vi "testing -- App - RUS scan V2.vi"(4 "Bypass error dialog":bool=TRUE, 5 "saved frequency unit":bool=TRUE, 6 "Zero amplitude at the end":bool, 7 "Save data settings":T3={"Save data"=TRUE, "Data Root Path"=path "C:/data/RUS/Experiment/ProbeTest/Probe10/YBCO_3/sweep4", "File Prefix"="289.47200K_1400_3000_", "File Format"=enum."BINARY", "Save column names"=FALSE, "File Comments"="<Description of the current file>\r\nColumns:Frequency\\tX\\tY\r\n    ITC Temp= 299.200000\r\n    LTC Temp= 0.000000\r\n          ITC_set=295.00000\r\n", "User/Prj"="<User Name/Project Description>"}, 8 "error in (no error)":errorcluster, 9 "Fast swep settings":T1={"Update rate (Hz)"=250.0, "Start F, Hz"=1400000.0, "Stop F"=3000000.0, "Number of points"=6000, "Amplitude"=2.1, "Init&amplitude"=TRUE, "IF"=1000.0, "Time constant"=0.003} {"IF" format="%#_6p"; "Amplitude" min=0.0 max=2.5; "Number of points" format="%.0p"; "Stop F" format="%#_6p"; "Start F, Hz" format="%#_6p"; "Update rate (Hz)" format="%0.2f"}, 11 "Lock-in DAQ settings":T2={"Lockin mode"=enum."NI-DAQ", "DAQmx Device"="Dev1", "SR Lockin"="GPIB0::10::INSTR", "Clock Multiplier"=64, "Low-pass filter"=enum."No filtering", "Ranges and couplings "=[{"Range"=2.5, "Coupling"=10106}], "Samples per read"=10, "Record IF"=FALSE, "Auto-phase"=FALSE} {"Ranges and couplings"."Coupling" items=["default"=-1, "RSE"=10083, "NRSE"=10078, "Differential"=10106, "Pseudodifferential"=12529]}) -> (0 "error out":errorcluster, 2 "Actual file path":path=path "C:/data/RUS/Experiment/ProbeTest/Probe10/YBCO_3/sweep4/February_2012/020712/289.73300K_1400_3000_001_020712.bin")   [LabVIEW 2010]
uses:
  <vilib>/Utility/error.llb/DialogType.ctl
  C:/Program Files (x86)/National Instruments/LabVIEW 2010/resource/objmgr/daqmx.rc
  RUS/Controls/Sweep settings.ctl
  RUS/Controls/Lock-in DAQ settings.ctl
  File/Controls/File formats.ctl
  File/Controls/Save data settings.ctl
  single sweep - adaptive parameters.ctl
  single sweep - frequency chunks.ctl
  wavepacket.ctl
  cursor winow.ctl
  next chunk -- parameters.ctl
  find peak -- parameters.ctl
panel:
  in  "Tab : everything":enum32{"main", "everything else", "adaptive"}(tab)=enum."adaptive"
  in  "complex plane scale gauge":dbl(slide)=0.07327431522473847 caption="Volts" scale=0.0001..0.1
  in  "show plot pallets":bool
  in  "highlight last # sec":dbl=4.0
  out "Plot:response":cluster{dbl[], dbl[]}[](graph)
  out "Plot:complex plane":cluster{dbl[], dbl[]}[](graph)
  in  "Tab : sweep controls":enum32{"Main controls", "File", "Advanced"}(tab)
  in  "Manual\nPhase":dbl(slide) scale=-180.0..180.0
  out "Error status byte\n(bit 5 - FAST aborted)":u8 format="%08b"
  out "STD status byte":u8 format="%08b"
  out "DO array  making time":u32=3
  out "DO write time, ms":u32=44
  out "Loop counter":i32=599
  out "Pre-sweep delay, s":dbl=0.2
  out "Samples in buffer":u32
  out "Actual setup time, ms":u32=1470
  in  "progress (sec)":dbl(slide)=0.20199999981559813 caption="seconds" min=80.0 max=80.0 scale=0.0..24.0
  in  "Plot when running":bool
  in  "algorithm":string="uniform"
  in  "Graph update rate, ms":u32=30
  in  "stop":bool
  out "Progress, %":u8(slide)=1 scale=0.0..100.0
  in  "cursor bracket: Scan, win":T5={"left"=1402.9280000000003, "right "=1414.9280000000003, "center"=1408.9280000000003, "window"=12.0, "cursors"=[1, 2, 3], "relative"=1, "absolute"=4, "fixed vertical offset"=2421.6740576496672, "vertical offset"=2421.6740576496672, "skew"=0.0, "default window frac"=0.0, "kind"=enum."symmetric", "skew.left"=0.5, "skew.right"=0.0, "Plot ref"=refnum, "wing order"=enum."back"}
  out "fancy circles":cluster{dbl[], dbl[]}[](array[cluster])=[{[0.004347976639836461, 0.0043237329011621035, 0.004251384023380436, 0.004132070991513198, 0.003967675443347089, 0.0037607899948818246, 0.0035146773532270816, 0.00323321886176232, 0.0029208532890330928, 0.002582506826719488, 0.00222351540065057, 0.0018495405200665291, 0.0014664799922359413, 0.001080374910511962, 0.0006973143826813736, 0.0003233395020973332, -3.56519239715844e-05, -0.0003739983862851902, -0.0006863639590144167, -0.0009678224504791784, -0.0012139350921339205, -0.0014208205405991845, -0.001585216088765295, -0.0017045291206325324, -0.0017768779984142003, -0.001801121737088557, -0.0017768779984142003, -0.0017045291206325324, -0.0015852160887652941, -0.001420820540599184, -0.00121393509213392, -0.000967822450479178, -0.0006863639590144162, -0.00037399838628518847, -3.5651923971582664e-05, 0.0003233395020973332, 0.0006973143826813741, 0.0010803749105119625, 0.0014664799922359426, 0.001849540520066531, 0.0022235154006505697, 0.002582506826719488, 0.0029208532890330936, 0.003233218861762321, 0.003514677353227083, 0.0037607899948818254, 0.003967675443347089, 0.004132070991513199, 0.004251384023380437, 0.0043237329011621035], [-0.00253283204245687, -0.0021474888509143563, -0.001768222751695333, -0.0014010149977470693, -0.0010516566747086093, -0.0007256573720308159, -0.00042815829345946126, -0.00016385117718095135, 6.309569569158376e-05, 0.0002491032374014545, 0.0003912379979003752, 0.0004872584271080889, 0.0005356502254961651, 0.0005356502254961651, 0.00048725842710808844, 0.0003912379979003752, 0.00024910323740145405, 6.309569569158376e-05, -0.00016385117718095135, -0.0004281582934594617, -0.0007256573720308154, -0.0010516566747086097, -0.00140101499774707, -0.0017682227516953328, -0.0021474888509143567, -0.002532832042456871, -0.002918175233999384, -0.003297441333218408, -0.003664649087166672, -0.004014007410205131, -0.004340006712882925, -0.004637505791454279, -0.004901812907732789, -0.005128759780605325, -0.005314767322315195, -0.005456902082814115, -0.0055529225120218295, -0.005601314310409906, -0.005601314310409906, -0.005552922512021829, -0.005456902082814115, -0.005314767322315195, -0.0051287597806053235, -0.004901812907732788, -0.004637505791454277, -0.004340006712882922, -0.004014007410205131, -0.0036646490871666704, -0.0032974413332184063, -0.0029181752339993822]}, {[-0.0007985969840225416, -0.0005913945404828922, -0.0003841920969432428, -0.0001769896534035934, 3.0212790136055923e-05, 0.00023741523367570524, 0.0004446176772153548, 0.0006518201207550041, 0.0008590225642946534, 0.0010662250078343027, 0.001273427451373952, 0.0014806298949136016, 0.001687832338453251, 0.0018950347819929002, 0.00210223722553255, 0.0023094396690721986, 0.002516642112611848, 0.0027238445561514977, 0.0029310469996911472, 0.003138249443230796], [-0.004804300169328853, -0.004577153356641655, -0.004350006543954456, -0.004122859731267258, -0.00389571291858006, -0.0036685661058928616, -0.003441419293205663, -0.003214272480518465, -0.0029871256678312666, -0.002759978855144068, -0.00253283204245687, -0.0023056852297696716, -0.002078538417082473, -0.0018513916043952751, -0.0016242447917080766, -0.0013970979790208786, -0.0011699511663336801, -0.0009428043536464817, -0.0007156575409592832, -0.0004885107282720852]}, {[-0.0009980406754980312, -0.0007708938628108329, -0.0005437470501236345, -0.0003166002374364362, -8.945342474923792e-05, 0.00013769338793796033, 0.0003648402006251588, 0.0005919870133123571, 0.0008191338259995553, 0.0010462806386867538, 0.0012734274513739518, 0.0015005742640611503, 0.0017277210767483488, 0.001954867889435547, 0.0021820147021227453, 0.0024091615148099433, 0.002636308327497142, 0.0028634551401843403, 0.0030906019528715387, 0.0033177487655587368], [-0.0004608076070603765, -0.0006680100506000258, -0.0008752124941396752, -0.0010824149376793247, -0.001289617381218974, -0.0014968198247586233, -0.0017040222682982728, -0.0019112247118379222, -0.0021184271553775715, -0.0023256295989172206, -0.00253283204245687, -0.0027400344859965196, -0.002947236929536169, -0.0031544393730758183, -0.003361641816615468, -0.003568844260155117, -0.0037760467036947664, -0.003983249147234416, -0.004190451590774065, -0.004397654034313714]}]
  out "window":cluster{dbl[], dbl[]}[](array[cluster])=[{array[500 elements], array[500 elements]}, {array[500 elements], array[500 elements]}, {[2988000.0, 2988320.0, 2988640.0, 2992640.0, 2996640.0, 3000640.0, 3004640.0, 3004960.0, 3008960.0, 3012960.0, 3013280.0, 3013600.0, 3017600.0, 3021600.0, 3025600.0, 3029600.0, 3033600.0, 3037600.0, 3041600.0, 3045600.0, 3049600.0, 3053600.0, 3057600.0, 3061600.0, 3065600.0, 3069600.0, 3073600.0, 3077600.0, 3077920.0, 3081920.0, 3085920.0, 3089920.0, 3093920.0, 3094240.0, 3098240.0, 3102240.0, 3102560.0, 3106560.0, 3110560.0, 3114560.0, 3118560.0, 3122560.0, 3126560.0, 3126880.0, 3130880.0, 1408320.0000000002, 1408640.0000000002, 1408960.0000000002, 1412960.0000000002, 1416960.0000000002], [0.00011132389559019453, 0.00010071650784182846, 0.00011473215051580125, 0.00014782978553753255, 0.00012363182181742826, 8.247818640394286e-05, 4.853569183607435e-05, 0.00011091209952173231, 5.335161099533373e-05, 8.997863187674346e-05, 6.096859045620223e-05, 0.00011032129342938127, 0.00014137261844608594, 0.00011027777124700277, 7.83124094059187e-05, 8.359930932665522e-05, 8.923138939621333e-05, 5.1551353463386254e-05, 8.295869472945261e-05, 8.128556971740557e-05, 7.69462000730066e-05, 7.144851315975473e-05, 7.952519321081926e-05, 9.517779850815267e-05, 9.704248606160299e-05, 0.00011632633414436816, 0.00010390576558171027, 0.00010696411213824573, 9.728970607203878e-05, 0.0001308279684608251, 6.464132471543712e-05, 0.00011952708368690759, 6.148514772660781e-05, 8.068062707804084e-05, 0.00011312139911462234, 6.908047023895298e-05, 5.936822230667681e-05, 0.00010020626764101784, 0.00012946703718681504, 0.00010013466000813908, 6.912354981532708e-05, 0.00011430443059521424, 0.00012513022719631484, 0.00010923915541343698, 0.00011547570124367561, 0.003905008531492904, 0.0033917347983675613, 0.003353407371274829, 0.003173893478063239, 0.003074549188462509]}, {[2988000.0, 2988320.0, 2988640.0, 2992640.0, 2996640.0, 3000640.0, 3004640.0, 3004960.0, 3008960.0, 3012960.0, 3013280.0, 3013600.0, 3017600.0, 3021600.0, 3025600.0, 3029600.0, 3033600.0, 3037600.0, 3041600.0, 3045600.0, 3049600.0, 3053600.0, 3057600.0, 3061600.0, 3065600.0, 3069600.0, 3073600.0, 3077600.0, 3077920.0, 3081920.0, 3085920.0, 3089920.0, 3093920.0, 3094240.0, 3098240.0, 3102240.0, 3102560.0, 3106560.0, 3110560.0, 3114560.0, 3118560.0, 3122560.0, 3126560.0, 3126880.0, 3130880.0, 1408320.0000000002, 1408640.0000000002, 1408960.0000000002, 1412960.0000000002, 1416960.0000000002], [0.013694694005932529, 0.014489837272950239, 0.009503558469975002, 0.009528211653947193, 0.012476459558180022, 0.013578618032833986, 0.020768560303619083, 0.020949019291147796, 0.02034486055557658, 0.011646926818591538, 0.009458678658119484, 0.006310537358577627, 0.00038583342676350336, 0.006103250811137311, 0.001250242454873757, 0.005243640192020321, 0.008719705117003948, 0.006143859432854482, 0.006470257084291946, 0.006348276391260311, 0.008375758813583493, 0.0038044691071716097, 0.0015818509944146705, 0.003581191521982118, 0.0006892804064302445, 0.0025054554152808646, 0.004117073317010084, 0.002045540413627015, 0.0007410657254269008, 0.005324792655608368, 0.012491486267365477, 0.013829845176253889, 0.009382411909246033, 0.008531253899751555, 0.006057094794442862, 0.000802518050976467, 0.006846069080773061, 0.004537353265510852, 0.008159903085244793, 0.0028444703551188284, 0.007454427723095375, 4.4410190171195404e-05, 0.0015101954709487865, 0.004475681662266171, 0.010341490132182555, 0.01226244459723875, 0.015308020505903021, 0.005597683037877003, 0.0037965342629815418, 0.0016913227005998597]}]
  in  "chunks":T6={"start F (Hz)"=1400000.0, "stop F (Hz)"=3000000.0, "total number of points"=6000, "chunk size"=10, "freq step (Hz)"=400.0, "update rate (Hz)"=250.0, "adaptive parameters"={"peaks are known -- parameters"={"Def Gamma (kHz)"=0.5, "dV"=15.0, "time in Gamma (sec)"=7.0, "phi-star"=0.0, "all peaks (kHz)"=[], "delta t (sec)"=22.0, "default step (Hz)"=0.0, "Max step (Hz)"=0.0, "all gamma (kHz)"=[564.0, 649.0, 987.0, 1133.0, 1214.0, 1585.0, 1763.0, 1823.0, 1880.0, 1899.0, 2032.0, 2138.0, 2221.0, 2270.0, 2350.0, 2456.0, 2580.0, 2634.0, 2831.0, 2960.0, 2965.0, 3131.0, 3328.0, 3469.0, 3553.0, 0.0, 3615.0, 3734.0, 0.0, 0.0, 0.0, 4236.0, 4300.0, 4331.0], "peaks OK"=FALSE, "gamma OK"=FALSE, "near omega (kHz)"=0.0, "near gamma (kHz)"=10000.0}, "find peak - parameters"={"wavepacket"={"R"=0.5, "wave number"=17.0, "delta k"=7.0, "radii vector"=[], "radial section"=[], "wave vector"=22.0, "wavepacket is"=TRUE}, "number of grid points"=70, "decimation threshold"=1, "Voltage range"=0.1, "target freq step"=20.0, "target spot size"=0.05, "factor"=1.0, "another factor"=1.0, "analyze last # sec"=3, "scale factor"=3}}, "total sweep time (sec)"=24.0, "chunk time (sec)"=0.04, "spot size (V)"=5.8152639158694506e-05, "uniform freq step (Hz)"=266.6666666666667, "next start freq (Hz)"=1412960.0000000002} {"next start freq (Hz)" format="%#9_8f"; "uniform freq step (Hz)" format="%#_3f"; "spot size (V)" format="%#_2f"; "adaptive parameters"."find peak - parameters"."wavepacket"."delta k" format="%#_3f"; "adaptive parameters"."find peak - parameters"."wavepacket"."wave number" format="%#_3f"; "adaptive parameters"."find peak - parameters"."wavepacket"."R" format="%#_3f"; "freq step (Hz)" format="%#4_4f"; "stop F (Hz)" format="%#_3f"; "start F (Hz)" format="%#_3f"}
  in  "adaptive parameters":T7={"peaks are known -- parameters"={"Def Gamma (kHz)"=0.5, "dV"=15.0, "time in Gamma (sec)"=7.0, "phi-star"=0.0, "all peaks (kHz)"=[], "delta t (sec)"=22.0, "default step (Hz)"=0.0, "Max step (Hz)"=0.0, "all gamma (kHz)"=[564.0, 649.0, 987.0, 1133.0, 1214.0, 1585.0, 1763.0, 1823.0, 1880.0, 1899.0, 2032.0, 2138.0, 2221.0, 2270.0, 2350.0, 2456.0, 2580.0, 2634.0, 2831.0, 2960.0, 2965.0, 3131.0, 3328.0, 3469.0, 3553.0, 0.0, 3615.0, 3734.0, 0.0, 0.0, 0.0, 4236.0, 4300.0, 4331.0], "peaks OK"=FALSE, "gamma OK"=FALSE, "near omega (kHz)"=0.0, "near gamma (kHz)"=10000.0}, "find peak - parameters"={"wavepacket"={"R"=0.5, "wave number"=17.0, "delta k"=7.0, "radii vector"=[], "radial section"=[], "wave vector"=22.0, "wavepacket is"=TRUE}, "number of grid points"=70, "decimation threshold"=1, "Voltage range"=0.1, "target freq step"=20.0, "target spot size"=0.05, "factor"=1.0, "another factor"=1.0, "analyze last # sec"=3, "scale factor"=3}} {"find peak - parameters"."wavepacket"."delta k" format="%#_3f"; "find peak - parameters"."wavepacket"."wave number" format="%#_3f"; "find peak - parameters"."wavepacket"."R" format="%#_3f"}
  out "Plot:window":cluster{dbl[], dbl[]}[](graph)
  # "SRS Lockin related"
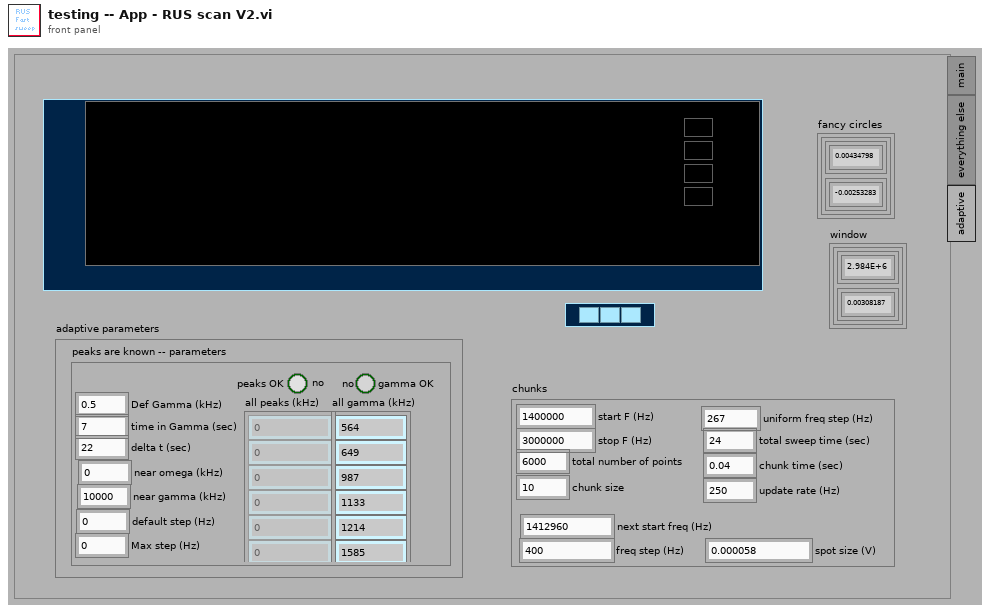
[diagram p1: front panel]
types:
  T1 = typedef "Sweep settings.ctl" = cluster{"Update rate (Hz)":dbl, "Start F, Hz":dbl, "Stop F":dbl, "Number of points":i32, "Amplitude":dbl, "Init&amplitude":bool, "IF":dbl, "Time constant":dbl}
  T2 = typedef "Lock-in DAQ settings.ctl" = cluster{"Lockin mode":enum16{"SRS", "NI-DAQ"}, "DAQmx Device":tag, "SR Lockin":refnum<visa-resource-name>, "Clock Multiplier":i32, "Low-pass filter":enum16{"No filtering", "Butterworth", "Bessel"}, "Ranges and couplings ":cluster{"Range":dbl, "Coupling":i32}[], "Samples per read":i32, "Record IF":bool, "Auto-phase":bool}
  T3 = typedef "Save data settings.ctl" = cluster{"Save data":bool, "Data Root Path":path, "File Prefix":string, "File Format":T4, "Save column names":bool, "File Comments":string, "User/Prj":string}
  T4 = typedef "File formats.ctl" = enum16{"TDMS", "ASCII", "BINARY"}
  T5 = typedef "cursor winow.ctl" = cluster{"left":dbl, "right ":dbl, "center":dbl, "window":dbl, "cursors":i32[], "relative":i32, "absolute":i32, "fixed vertical offset":dbl, "vertical offset":dbl, "skew":dbl, "default window frac":dbl, "kind":enum16{"symmetric", "skewed", "fancy"}, "skew.left":dbl, "skew.right":dbl, "Plot ref":refnum<vi>, "wing order":enum16{"forw", "back"}}
  T6 = typedef "single sweep - frequency chunks.ctl" = cluster{"start F (Hz)":dbl, "stop F (Hz)":dbl, "total number of points":i32, "chunk size":i32, "freq step (Hz)":dbl, "update rate (Hz)":dbl, "adaptive parameters":T7, "total sweep time (sec)":dbl, "chunk time (sec)":dbl, "spot size (V)":dbl, "uniform freq step (Hz)":dbl, "next start freq (Hz)":dbl}
  T7 = typedef "single sweep - adaptive parameters.ctl" = cluster{"peaks are known -- parameters":T8, "find peak - parameters":T9}
  T8 = typedef "next chunk -- parameters.ctl" = cluster{"Def Gamma (kHz)":dbl, "dV":dbl, "time in Gamma (sec)":dbl, "phi-star":dbl, "all peaks (kHz)":dbl[], "delta t (sec)":dbl, "default step (Hz)":dbl, "Max step (Hz)":dbl, "all gamma (kHz)":dbl[], "peaks OK":bool, "gamma OK":bool, "near omega (kHz)":dbl, "near gamma (kHz)":dbl}
  T9 = typedef "find peak -- parameters.ctl" = cluster{"wavepacket":T10, "number of grid points":i32, "decimation threshold":i32, "Voltage range":dbl, "target freq step":dbl, "target spot size":dbl, "factor":dbl, "another factor":dbl, "analyze last # sec":i32, "scale factor":i32}
  T10 = typedef "wavepacket.ctl" = cluster{"R":dbl, "wave number":dbl, "delta k":dbl, "radii vector":dbl[], "radial section":cdb[], "wave vector":dbl, "wavepacket is":bool}
  T11 = typedef "RUS settings.ctl" = cluster{"NI-DAQ lockin settings":T12, "Fast swep settings":T1, "Pre-sweep delay, s":dbl, "Lockin mode":enum16{"SRS", "NI-DAQ"}, "SR Lockin":refnum<visa-resource-name>, "DAQmx Device":tag, "Clock Multiplier":i32, "Fast Sweep Data Out":cluster{"DO clock task":refnum<k21>, "DO task":refnum<k21>, "Update clock task":refnum<k21>, "DAQ lockin task":refnum<k21>, "Pre-sweep counter task":refnum<k21>}, "Lockin Range, V":sgl, "F Array":dbl[], "Freq. update clock terminal":string, "DO Clock Rate (Hz)":dbl, "ADC clock terminal":string, "Pre-sweep counter terminal":string, "Samples per read":i32, "DO clock terminal":string, "Pre-sweep points":i32, "F points per write":i32, "Total sweep time, s":dbl, "Initial SYNTH phase":dbl, "Record IF":bool, "Save data settings":T3, "Data file path":path, "New data user event":refnum<user-event>, "Stop user event":refnum<user-event>, "Number of channels":i32, "Auto-phase":bool}
  T12 = typedef "RUS NI-DAQ Lockin Settings.ctl" = cluster{"Samples per sine wave":i32, "Sine waves per freq step":i32, "Output Representation":enum16{"Real/Imaginary", "Polar"}, "Low-pass filter":enum16{"No filtering", "Butterworth", "Bessel"}, "Ranges and couplings ":cluster{"Range":dbl, "Coupling":i32}[]}
  T13 = enum16{"", "cursor moves", "center change", "window change", "init", "check", "reset", "set y to middle"}
  T14 = typedef "LVCursorListTypeDef.ctl" = cluster{"Name":string, "Color":u32, "Style":u8, "Point Style":u8, "Name Visible":bool, "Allow Drag":bool, "Cursor Mode":u32, "Plot":i32, "Index":i32, "Position":cluster{"X":dbl, "Y":dbl}, "X Scale":u32, "Y Scale":u32, "Watch Plots":i32[], "Watch All Plots":bool, "Plot Area":i32, "Label Offset":cluster{"X":dbl, "Y":dbl}}[]
  T15 = cluster{"left":dbl, "right ":dbl, "center":dbl, "window":dbl, "cursors":i32[], "relative":i32, "absolute":i32, "fixed vertical offset":dbl, "vertical offset":dbl, "skew":dbl, "default window frac":dbl, "kind":enum16{"symmetric", "skewed", "fancy"}, "skew.left":dbl, "skew.right":dbl, "Plot ref":refnum<vi>, "wing order":enum16{"forw", "back"}}
  T16 = typedef "DialogType.ctl" = u16
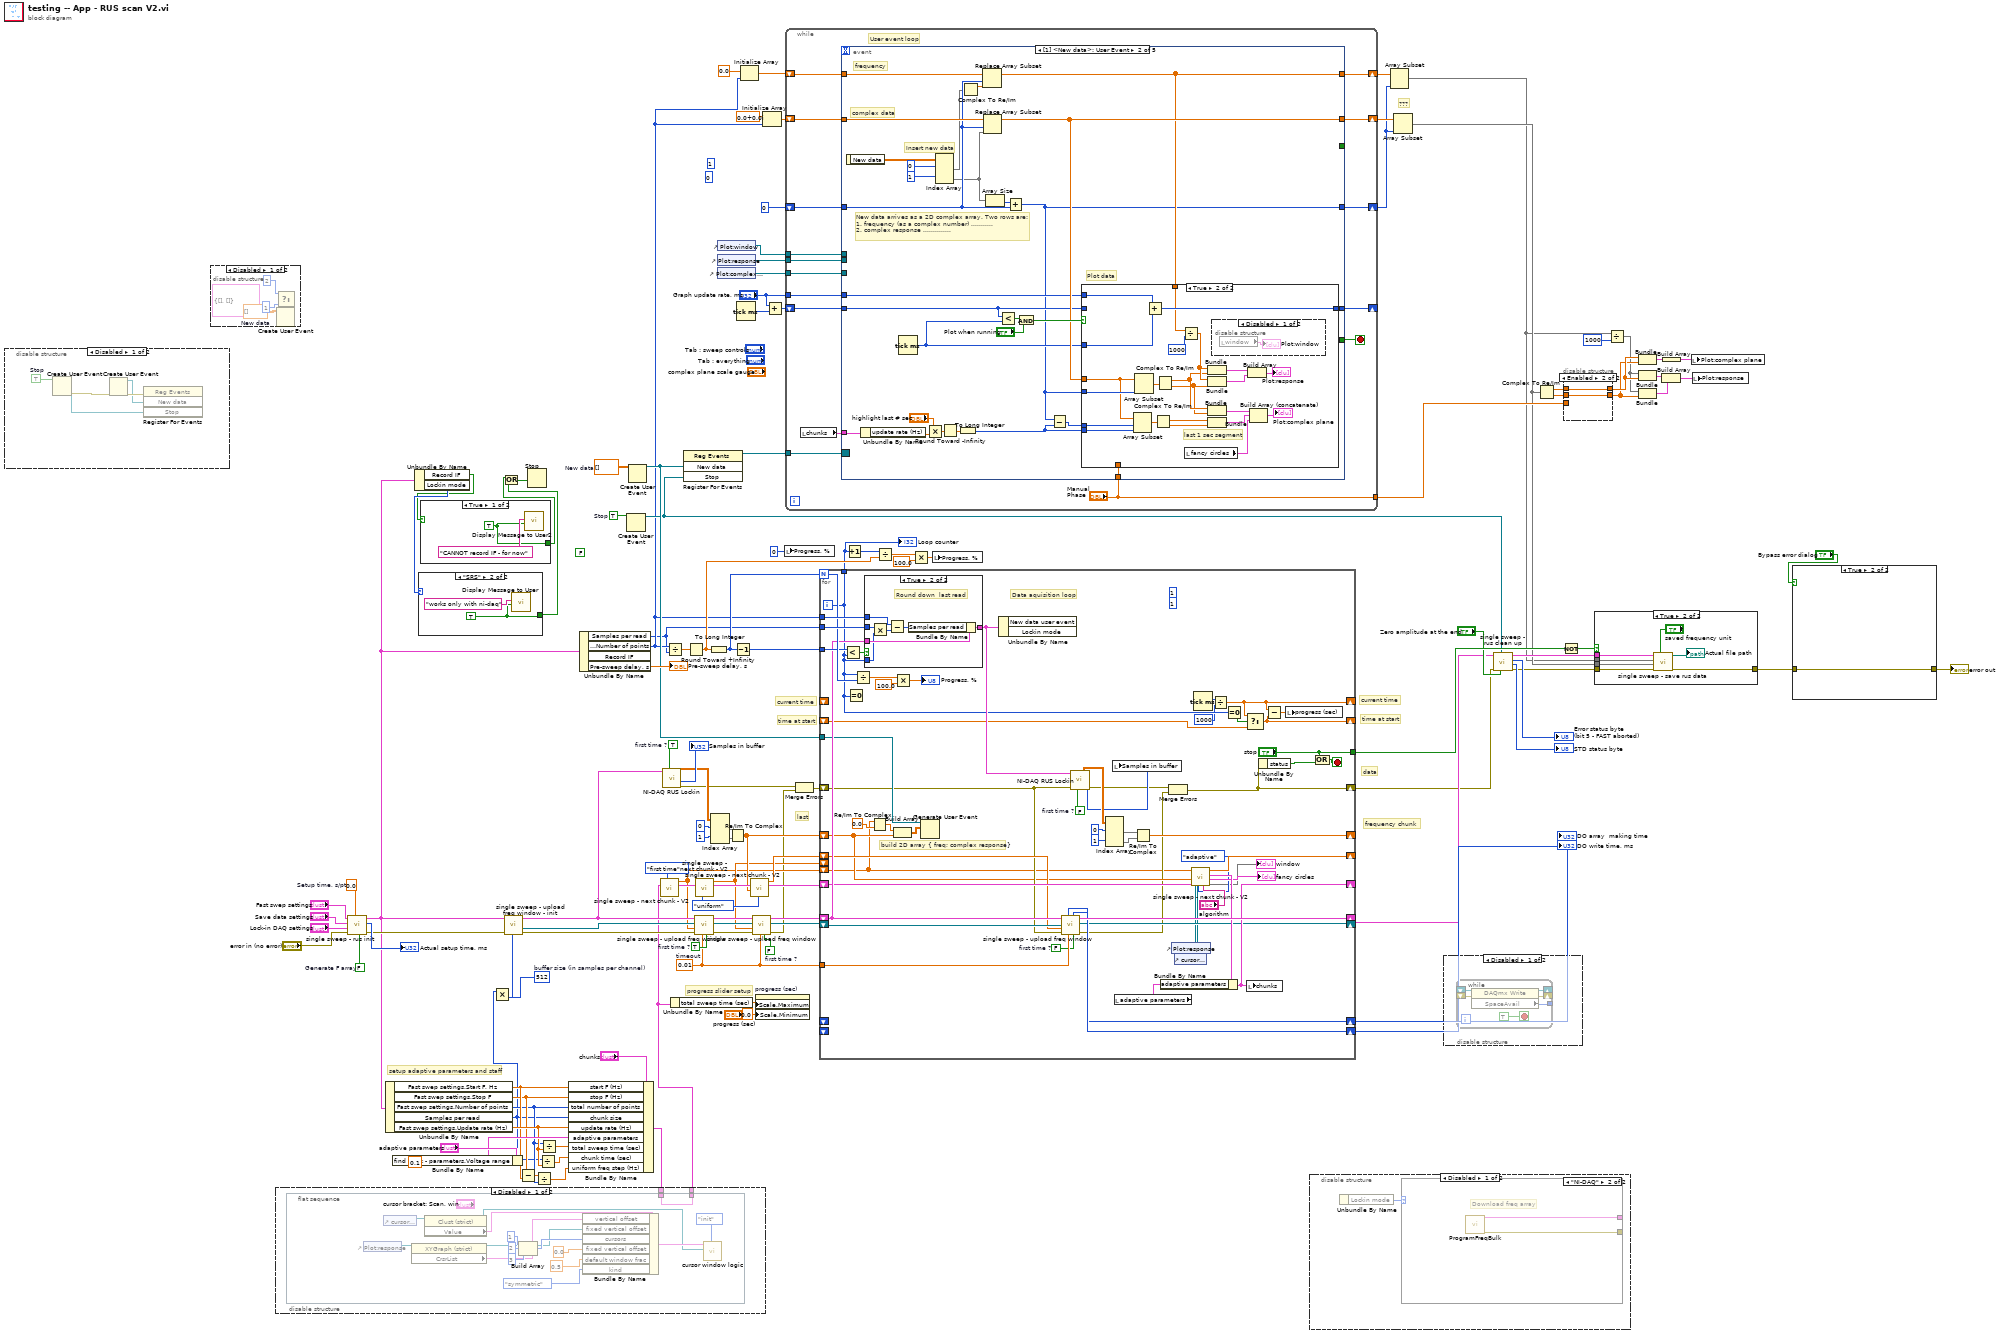
[diagram p0: block diagram]
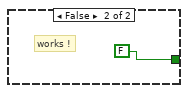
[diagram p4: hidden frame]
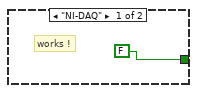
[diagram p7: hidden frame]
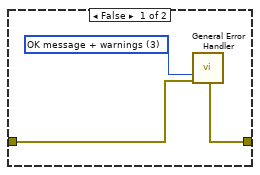
[diagram p10: hidden frame]
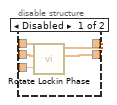
[diagram p11: hidden frame]
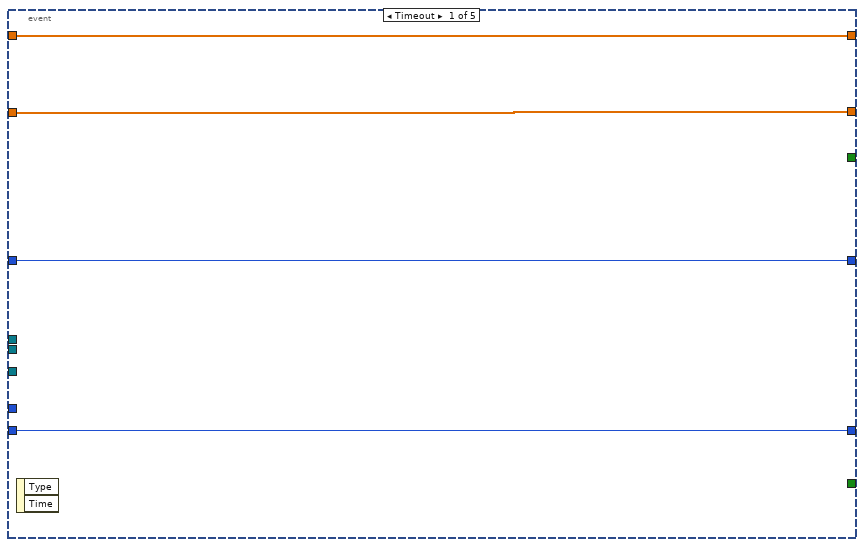
[diagram p12: hidden frame]
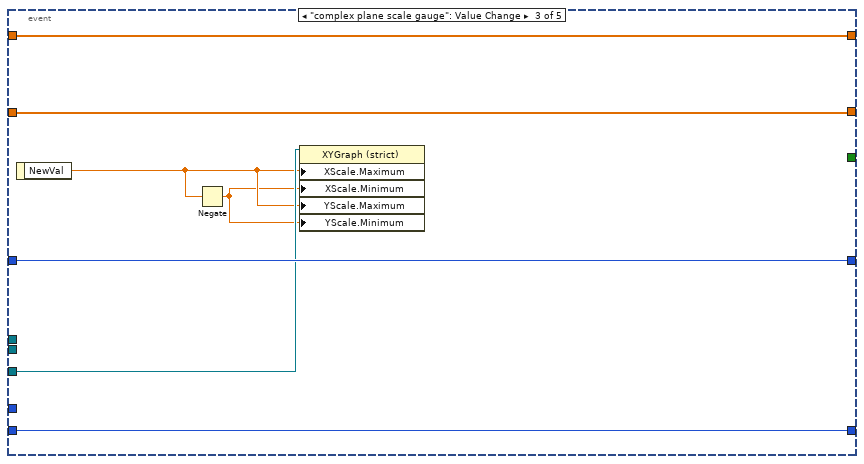
[diagram p15: hidden frame]
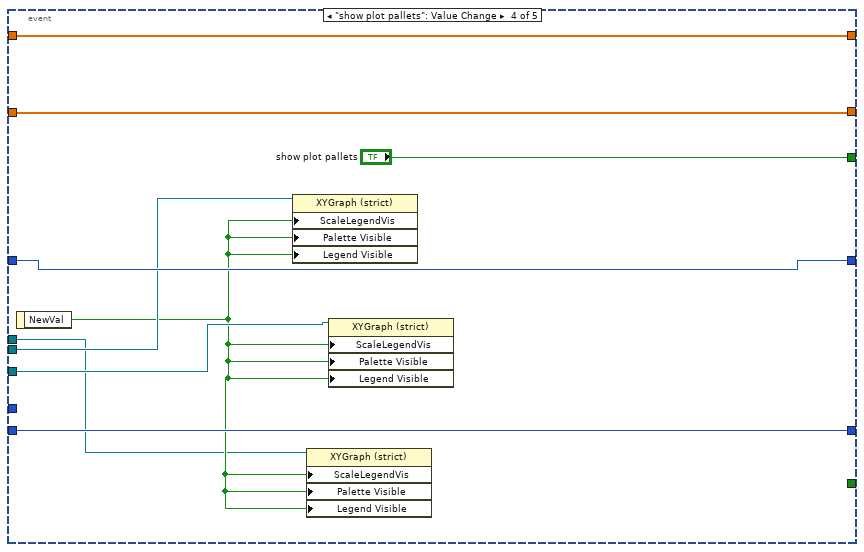
[diagram p16: hidden frame]
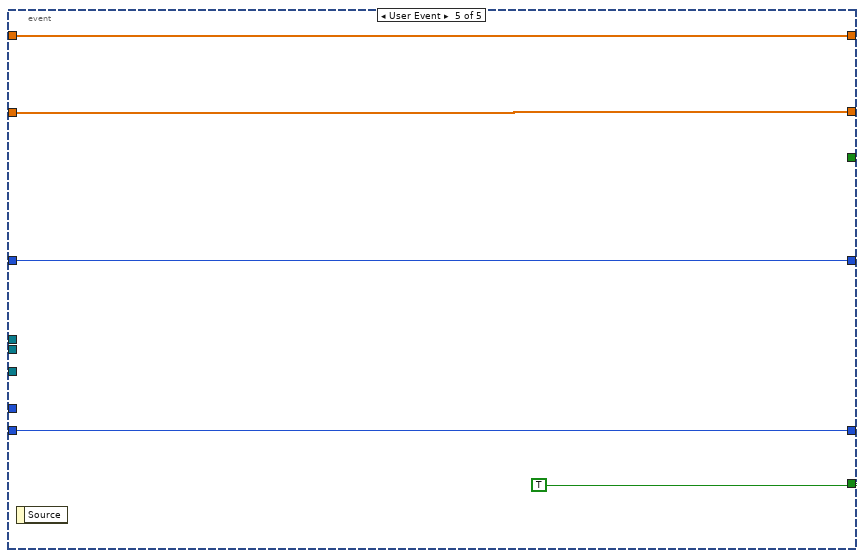
[diagram p17: hidden frame]
diagram:
  w11 = TRUE  # first time ?
  w12 = FALSE  # Generate F array
  w13 = 0.0  # Setup time, s/pt
  w16 = u32 512  # buffer size (in samples per channel)
  w33 = FALSE  # first time ?
  (unwired) 0 ("disabled index (col)")
  (unwired) FALSE
  (unwired) 1 ("dimension size")
  w77 = cdb[][] []  # New data
  w80 = TRUE  # Stop
  w19 = enum16{"first time", "uniform", "adaptive"}."uniform" ("mode")
  w85 = TRUE  # first time ?
  w26 = 0.01  # timeout
  # "data"
  # "frequency chunk"
  # "last"
  # "setup adaptive parameters and staff"
  # "time at start"
  # "current time"
  # "time at start"
  # "current time"
  # "progress slider setup"
  # "???"
  n1 = disable-structure shown="Disabled" {
    frame Disabled {
      w129 = TRUE  # Stop
      n2 = Create User Event(user event datatype=w129) -> (user event=w126:refnum<user-event>, error out=w128:errorcluster)  [unwired: 1 in]
      n3 = Create User Event(error in=w128) -> (user event datatype=w124:cluster{}, user event=w125:refnum<user-event>, error out=w127:errorcluster)
      n4 = register-events(error in=w127, w125, w126) -> ()  [unwired: 1 in, 2 out]
    }
    frame Enabled {
    }
  }
  n5 = disable-structure shown="Disabled" {
    frame Disabled {
      w130 = cdb[][] []  # New data
      (unwired) cluster{cdb[], dbl[]} {[], []} ("Newer data")
      n6 = Create User Event(user event datatype=w130) -> ()  [unwired: 1 in, 2 out]
      n7 = Select(t=2 ("dimension size"), f=1 ("dimension size")) -> ()  [unwired: 1 in, 1 out]
    }
    frame Enabled {
    }
  }
  n8 = call "single sweep - rus init.vi"("Generate F array"=w12, "Setup time, s/pt"=w13, "error in (no error)"="error in (no error)", "Lock-in DAQ settings"="Lock-in DAQ settings", "Save data settings"="Save data settings", "Fast swep settings"="Fast swep settings") -> ("error out"=w89:errorcluster, "Actual setup time, ms"=→"Actual setup time, ms":u32, "RUS settings out"=w78:T11)  [unwired: 2 in, 1 out]
  n9 = Unbundle By Name(w78) -> ("Fast swep settings.Start F, Hz"=w40:dbl, "Fast swep settings.Stop F"=w39:dbl, "Fast swep settings.Number of points"=w37:i32, "Samples per read"=w14:i32, "Fast swep settings.Update rate (Hz)"=w54:dbl)
  n10 = Bundle By Name(cluster="adaptive parameters", "find peak - parameters.Voltage range"=0.1 ("Voltage Span")) -> (w56:T7)
  n11 = Unbundle By Name(w78) -> ("Record IF"=w49:bool, "Lockin mode"=w88:enum16{"SRS", "NI-DAQ"})
  n12 = case shown="\"SRS\"" w88 {
    tunnel: [FALSE w134] -> w51
    frame "NI-DAQ" {
      # "works !"
    }
    frame "SRS" {
      w134 = TRUE
      n13 = call "Display Message to User"("Enable"=w134, "Message"="works only with ni-daq") -> ()  [unwired: 8 in, 2 out]
    }
  }
  n14 = case shown="True" w49 {
    tunnel: [w136 FALSE] -> w50
    frame True {
      w136 = TRUE
      n15 = call "Display Message to User2"("Enable"=w136, "Message"="CANNOT record IF - for now") -> ()  [unwired: 8 in, 2 out]
    }
    frame False {
      # "works !"
    }
  }
  n16 = Multiply(x=w14, y=w16) -> (x*y=w15:u32)
  n17 = Or(x=w50, y=w51) -> (x .or. y?=w48:bool)
  n18 = call "single sweep - upload freq window - init.vi"("buffer size (in samples per channel)"=w15, "error in (no error)"=w89, "RUS settings"=w78) -> ("error - out"=w22:errorcluster, "task out"=w87:refnum<k21>, "RUS settings out"=w34:T11)  [unwired: 6 in]
  n19 = Subtract(x=w39, y=w40) -> (x-y=w38:dbl)
  n20 = Stop(stop? (T)=w48) -> ()
  n21 = Divide(x=w38, y=w37) -> (x/y=w36:dbl)
  n22 = Divide(x=w14, y=w54) -> (x/y=w52:dbl)
  n23 = Divide(x=w37, y=w54) -> (x/y=w53:dbl)
  n24 = Bundle By Name(cluster="chunks", "start F (Hz)"=w40, "stop F (Hz)"=w39, "total number of points"=w37, "chunk size"=w14, "update rate (Hz)"=w54, "adaptive parameters"=w56, "total sweep time (sec)"=w53, "chunk time (sec)"=w52, "uniform freq step (Hz)"=w36) -> (w2:T6)
  n25 = disable-structure shown="Disabled" {
    disable-tunnel: w2 -> [w140 w157]
    disable-tunnel: [w139 w157] -> w1
    frame Disabled {
      n26 = flat-sequence {
        tunnel: [w141] -> w139
        tunnel: w140 -> [w141]
        frame #0 {
          n27 = control-ref of="Plot:response"() -> (w144:refnum<vi>)
          n28 = control-ref of="cursor bracket: Scan, win"() -> (w145:refnum<vi>)
          n29 = property on="Property Node" class="XYGraph (strict)"(reference=w144) -> (reference out=w143:refnum<vi>, "CrsrList"=w142:T14)  [unwired: 1 in, 1 out]
          n30 = property class="Clust (strict)"(reference=w145) -> (reference out=w147:refnum<vi>, "Value"=w146:T15)  [unwired: 1 in, 1 out]
          n31 = Build Array(1, 2, 3) -> (w155:i32[])
          n32 = Bundle By Name(cluster=w146, "vertical offset"=w142, "fixed vertical offset"=w143, "cursors"=w155, "fixed vertical offset"=0.0, "default window frac"=0.5 ("fixed vertical offset"), "kind"=enum16{"symmetric", "skewed", "fancy"}."symmetric") -> (w156:T15)
          n33 = call "cursor window logic.vi"("cursor window action"=T13."init" ("action"), 10:"cursor bracket in"=w147, 11:"cursor bracket in"=w156) -> ()  [unwired: 7 in, 2 out]
        }
      }
    }
    frame Enabled {
    }
  }
  n34 = Unbundle By Name(w78) -> ("Samples per read"=w41:i32, "Fast swep settings.Number of points"=w42:i32, "Pre-sweep delay, s"=→"Pre-sweep delay, s":dbl)  [unwired: 1 out]
  n35 = Create User Event(user event datatype=w80) -> (user event=w64:refnum<user-event>)  [unwired: 1 in, 1 out]
  n36 = Create User Event(user event datatype=w77) -> (user event=w79:refnum<user-event>)  [unwired: 1 in, 1 out]
  n37 = call "single sweep - next chunk - V2.vi"("mode"=enum16{"first time", "uniform", "adaptive"}."first time", "chunks"=w1) -> ("chunks out"=w86:T6, "F Array"=w17:dbl[])  [unwired: 7 in, 1 out]
  n38 = call "NI-DAQ RUS Lockin.vi"("Init?"=w11, "RUS settings"=w34) -> ("error out"=w4:errorcluster, "AvailSampPerChan"=→"Samples in buffer":u32, "Lockin out"=w5:dbl[][])  [unwired: 6 in, 1 out]
  n39 = Divide(x=w42, y=w41) -> (x/y=w121:dbl)
  n40 = Unbundle By Name(w1) -> ("total sweep time (sec)"=w47:dbl)
  n41 = register-events(w79, w64) -> (reference out=w81:refnum<event-registration>)  [unwired: 2 in, 1 out]
  n42 = Round Toward +Infinity(x=w121) -> (ceil(x): smallest int >= x=w115:dbl)
  n43 = call "single sweep - upload freq window.vi"("first time ?"=w85, "timeout"=w26, "error in (no error)"=w22, "F-window array"=w17, "task in"=w87, "RUS settings"=w34) -> ("error out"=w21:errorcluster, "task out"=w29:refnum<k21>, "RUS settings out"=w32:T11)  [unwired: 1 in, 2 out]
  n44 = call "single sweep - next chunk - V2.vi"("mode"=w19, "chunks"=w86) -> ("chunks out"=w28:T6, "F Array"=w18:dbl[])  [unwired: 7 in, 1 out]
  n45 = To Long Integer(number=w115) -> (32bit integer=w99:i32)
  n46 = Index Array(array=w5, index (row) #1=0 ("index"), index (row) #2=1 ("length")) -> (element #1=w7:dbl[], element #2=w6:dbl[])  [unwired: 2 in]
  n47 = control-ref of="Plot:window"() -> (w35:refnum<vi>)
  n48 = control-ref of="Plot:response"() -> (w60:refnum<vi>)
  n49 = control-ref of="Plot:complex plane"() -> (w59:refnum<vi>)
  n50 = Re/Im To Complex(1:w6, 2:w7) -> (0:w20:cdb[])
  n51 = Decrement(x=w99) -> (x-1=w111:i32)
  n52 = Tick Count (ms)() -> (millisecond timer value=w122:u32)
  n53 = Initialize Array(0.0 ("Numeric"), w42) -> (w73:dbl[])
  n54 = call "single sweep - next chunk - V2.vi"("mode"=w19, "x + iy"=w20, "chunks"=w28) -> ("chunks out"=w27:T6, "F Array"=w24:dbl[])  [unwired: 6 in, 1 out]
  n55 = call "single sweep - upload freq window.vi"("first time ?"=w33, "timeout"=w26, "error in (no error)"=w21, "F-window array"=w18, "task in"=w29, "RUS settings"=w32) -> ("error out"=w3:errorcluster, "task out"=w30:refnum<k21>, "RUS settings out"=w31:T11)  [unwired: 1 in, 2 out]
  n56 = property on="progress (sec)" class="Slide (strict)"("Scale.Maximum"=w47, "Scale.Minimum"=0.0 ("Data Entry Limits:Minimum")) -> ()  [unwired: 2 in, 2 out]
  n57 = Initialize Array(cdb 0.0+0.0i ("Numeric"), w42) -> (w113:cdb[])
  n58 = Add(x="Graph update rate, ms", y=w122) -> (x+y=w92:u32)
  n59 = local write "Progress, %"(u8 0 ("Progress")) -> ()
  n60 = while {
    tunnel: w81 -> [w173]
    shift-right: [w171] -> w106
    shift-left: w113 -> [w170]
    shift-right: [w167] -> _
    shift-left: w92 -> [w169]
    tunnel: "Graph update rate, ms" -> [w168]
    shift-right: [w165] -> w61
    shift-left: 0 ("disabled index (col)") -> [w166]
    tunnel: ["Manual\nPhase"] -> w103
    shift-right: [w162] -> w62
    shift-left: w73 -> [w164]
    tunnel: w60 -> [w161]
    tunnel: w59 -> [w160]
    tunnel: w35 -> [w158]
    stop <- w172 stop-if-true
    # "User event loop"
    n61 = local read "chunks"() -> (w159:T6)
    n62 = event shown="[1] <New data>: User Event" {
      selector: w173 -> [_ _ _ _ _]
      dyn-events: _ -> [_ _ _ _ _]
      timeout: _ -> [_ _ _ _ _]
      tunnel: [_ _ _ _ TRUE] -> w172
      tunnel: [w177 w202 w236 w245 w250] -> w171
      tunnel: w170 -> [w177 w203 w236 w245 w250]
      tunnel: w169 -> [w176 w198 w235 w244 w249]
      tunnel: w168 -> [_ w196 _ _ _]
      tunnel: [w176 w205 w235 w244 w249] -> w167
      tunnel: w166 -> [w175 w190 w234 w243 w248]
      tunnel: [w175 w183 w234 w243 w248] -> w165
      tunnel: w164 -> [w174 w192 w237 w246 w247]
      tunnel: "Manual\nPhase" -> [_ w201 _ _ _]
      tunnel: [w174 w191 w237 w246 w247] -> w162
      tunnel: w161 -> [_ _ _ w242 _]
      tunnel: w160 -> [_ _ w233 w241 _]
      tunnel: [_ _ _ "show plot pallets" _] -> _
      tunnel: w159 -> [_ w186 _ _ _]
      tunnel: w158 -> [_ _ _ w238 _]
      event Timeout {
        n63 = event-data() -> ()  [unwired: 3 out]
      }
      event User Event {
        # "complex data"
        # "frequency"
        # "Plot data"
        # "New data arrives as a 2D complex array. Two rows are: \n1. frequency (as a complex number) ........... \n2. complex response .............."
        # "Insert new data"
        n64 = event-data() -> ("New data"=w195:cdb[][])  [unwired: 1 out]
        n65 = Unbundle By Name(w186) -> ("update rate (Hz)"=w185:dbl)
        n66 = Tick Count (ms)() -> (millisecond timer value=w197:u32)
        n67 = Multiply(x="highlight last # sec", y=w185) -> (x*y=w184:dbl)
        n68 = Index Array(array=w195, index (row) #1=0 ("disabled index (col)"), index (row) #2=1 ("disabled index (col)")) -> (element #1=w189:cdb[], element #2=w181:cdb[])  [unwired: 2 in]
        n69 = Round Toward -Infinity(1:w184) -> (0:w179:dbl)
        n70 = To Long Integer(number=w179) -> (32bit integer=w178:i32)
        n71 = Complex To Re/Im(x + iy=w189) -> (x=w188:dbl[])  [unwired: 1 out]
        n72 = Replace Array Subset(array=w192, new element=w188, index=w190) -> (w191:dbl[])
        n73 = Replace Array Subset(array=w203, new element=w181, index=w190) -> (w202:cdb[])
        n74 = Array Size(array=w181) -> (size(s)=w180:i32)
        n75 = Less?(x=w198, y=w197) -> (x < y?=w200:bool)
        n76 = Add(x=w180, y=w190) -> (x+y=w183:i32)
        n77 = And(x=w200, y="Plot when running") -> (x .and. y?=w204:bool)
        n78 = Subtract(x=w183, y=w178) -> (x-y=w182:i32)
        n79 = case shown="True" w204 {
          tunnel: w202 -> [_ w216]
          tunnel: w197 -> [_ w225]
          tunnel: [w206 w224] -> w205
          tunnel: w198 -> [w206 _]
          tunnel: w191 -> [_ w212]
          tunnel: w183 -> [_ w222]
          tunnel: w201 -> [_ _]
          tunnel: w196 -> [_ w226]
          tunnel: w182 -> [_ w218]
          tunnel: w178 -> [_ w217]
          frame False {
          }
          frame True {
            # "last 1 sec segment"
            n80 = Array Subset(array=w216, index=w218, length=w217) -> (w219:cdb[])
            n81 = Array Subset(array=w216, length=w222) -> (w221:cdb[])  [unwired: 1 in]
            n82 = Add(x=w226, y=w225) -> (x+y=w224:u32)
            n83 = Complex To Re/Im(x + iy=w219) -> (x=w215:dbl[], y=w214:dbl[])
            n84 = Complex To Re/Im(x + iy=w221) -> (x=w209:dbl[], y=w208:dbl[])
            n85 = Divide(x=w212, y=1000 ("dimension size")) -> (x/y=w211:dbl[])
            n86 = local read "fancy circles"() -> (w207:cluster{dbl[], dbl[]}[])
            n87 = Bundle(w211, w209) -> (w229:cluster{dbl[], dbl[]})  [unwired: 1 out]
            n88 = Bundle(w211, w208) -> (w227:cluster{dbl[], dbl[]})  [unwired: 1 out]
            n89 = Bundle(w209, w208) -> (w220:cluster{dbl[], dbl[]})  [unwired: 1 out]
            n90 = Bundle(w215, w214) -> (w213:cluster{dbl[], dbl[]})  [unwired: 1 out]
            n91 = disable-structure shown="Disabled" {
              frame Disabled {
                n92 = local read "window"() -> (→"Plot:window":cluster{dbl[], dbl[]}[])
              }
              frame Enabled {
              }
            }
            n93 = Build Array(w229, w227) -> (→"Plot:response":cluster{dbl[], dbl[]}[])
            n94 = Build Array (concatenate)(w220, w213, w207) -> (→"Plot:complex plane":cluster{dbl[], dbl[]}[])
          }
        }
      }
      event "complex plane scale gauge": Value Change {
        n95 = event-data() -> ("NewVal"=w232:dbl)  [unwired: 1 out]
        n96 = Negate(x=w232) -> (-x=w231:dbl)
        n97 = property on="Property Node" class="XYGraph (strict)"(reference=w233, "XScale.Maximum"=w232, "XScale.Minimum"=w231, "YScale.Maximum"=w232, "YScale.Minimum"=w231) -> ()  [unwired: 1 in, 2 out]
      }
      event "show plot pallets": Value Change {
        n98 = event-data() -> ("NewVal"=w239:bool)  [unwired: 1 out]
        n99 = property on="Property Node" class="XYGraph (strict)"(reference=w242, "ScaleLegendVis"=w239, "Palette Visible"=w239, "Legend Visible"=w239) -> ()  [unwired: 1 in, 2 out]
        n100 = property on="Property Node" class="XYGraph (strict)"(reference=w238, "ScaleLegendVis"=w239, "Palette Visible"=w239, "Legend Visible"=w239) -> ()  [unwired: 1 in, 2 out]
        n101 = property on="Property Node" class="XYGraph (strict)"(reference=w241, "ScaleLegendVis"=w239, "Palette Visible"=w239, "Legend Visible"=w239) -> ()  [unwired: 1 in, 2 out]
      }
      event User Event {
        n102 = event-data() -> ()  [unwired: 2 out]
      }
    }
  }
  n103 = Merge Errors(w4, w3) -> (w25:errorcluster)
  n104 = for {
    N: w99 -> [w304]
    tunnel: w41 -> [w306]
    tunnel: [w275] -> w114
    tunnel: w111 -> [w300]
    tunnel: w42 -> [w307]
    tunnel: ["stop"] -> w105
    shift-right: [w295] -> w63
    shift-left: w31 -> [w297]
    tunnel: w26 -> [w296]
    shift-right: [w290] -> w84
    shift-left: _ -> [_]
    shift-right: [w257] -> _
    shift-left: w30 -> [w292]
    shift-right: [w260] -> w23
    shift-left: w25 -> [w261]
    shift-right: [w294] -> _
    shift-left: w24 -> [w262]
    shift-right: [w278] -> _
    shift-left: w27 -> [w293]
    shift-right: [w291] -> w83
    shift-left: _ -> [_]
    tunnel: w79 -> [w288]
    shift-right: [w269] -> _
    shift-left: _ -> [_]
    shift-right: [w268] -> _
    shift-left: _ -> [w270]
    shift-right: [w263] -> _
    shift-left: w20 -> [w259]
    shift-left: w18 -> [_]
    shift-left: w17 -> [w255]
    i -> [w275]
    stop <- w309 stop-if-true
    w264 = FALSE  # first time ?
    (unwired) 1 ("length")
    (unwired) 1 ("index")
    w289 = FALSE  # first time ?
    # "build 2D array { freq; complex response}"
    # "Data aquisition loop"
    n105 = Less?(x=w300, y=w275) -> (x < y?=w308:bool)
    n106 = Equal To 0?(x=w275) -> ()  [unwired: 1 out]
    n107 = Divide(x=w275, y=w304) -> (x/y=w303:dbl)
    n108 = case shown="True" w308 {
      tunnel: w307 -> [_ w317]
      tunnel: w306 -> [_ w312]
      tunnel: w275 -> [_ w311]
      tunnel: w297 -> [w310 w315]
      tunnel: [w310 w313] -> w305
      frame False {
      }
      frame True {
        # "Round down  last read"
        n109 = Multiply(x=w312, y=w311) -> (x*y=w316:i32)
        n110 = Subtract(x=w317, y=w316) -> (x-y=w314:i32)
        n111 = Bundle By Name(cluster=w315, "Samples per read"=w314) -> (w313:T11)
      }
    }
    n112 = Re/Im To Complex(1:0.0, 2:w255) -> (0:w281:cdb[])
    n113 = Build Array(w281, w259) -> (w280:cdb[][])
    n114 = Multiply(x=w303, y=100.0) -> (x*y=→"Progress, %":dbl)
    n115 = Generate User Event(user event=w288, event data cluster=w280) -> ()  [unwired: 1 in, 2 out]
    n116 = Unbundle By Name(w305) -> ()  [unwired: 2 out]
    n117 = call "single sweep - upload freq window.vi"("first time ?"=w289, "timeout"=w296, "error in (no error)"=w261, "F-window array"=w262, "task in"=w292, "RUS settings"=w297) -> ("error out"=w256:errorcluster, "task out"=w257:refnum<k21>, "RUS settings out"=w295:T11, "DO array  making time"=w290:u32, "DO write time"=w291:u32)  [unwired: 1 in]
    n118 = call "NI-DAQ RUS Lockin.vi"("Init?"=w264, "error in (no error)"=w261, "RUS settings"=w305) -> ("error out"=w258:errorcluster, "AvailSampPerChan"=w265:u32, "Lockin out"=w287:dbl[][])  [unwired: 5 in, 1 out]
    n119 = Index Array(array=w287, index (row) #1=0 ("index"), index (row) #2=1 ("length")) -> (element #1=w284:dbl[], element #2=w283:dbl[])  [unwired: 2 in]
    n120 = local write "Samples in buffer"(w265) -> ()
    n121 = local read "adaptive parameters"() -> (w277:T7)
    n122 = Re/Im To Complex(1:w283, 2:w284) -> (0:w263:cdb[])
    n123 = Merge Errors(w258, w256) -> (w260:errorcluster)
    n124 = control-ref of="Plot:response"() -> (w253:refnum<vi>)
    n125 = control-ref of="cursor bracket: Scan, win"() -> (w252:refnum<vi>)
    n126 = call "single sweep - next chunk - V2.vi"("algorithm"="algorithm", 5:w252, "mode"=enum16{"first time", "uniform", "adaptive"}."adaptive", 7:w253, "x + iy"=w259, "chunks"=w293, "F Array in"=w255) -> (0:→"window", "fancy circles"=→"fancy circles":cluster{dbl[], dbl[]}[], "chunks out"=w279:T6, "F Array"=w294:dbl[])  [unwired: 1 in]
    n127 = Bundle By Name(cluster=w279, "adaptive parameters"=w277) -> (w278:T6)
    n128 = Tick Count (ms)() -> (millisecond timer value=w274:u32)
    n129 = Divide(x=w274, y=u32 1000) -> (x/y=w269:dbl)
    n130 = Equal To 0?(x=w275) -> (x = 0?=w271:bool)
    n131 = Select(t=w269, s=w271, f=w270) -> (s? t:f=w268:dbl)
    n132 = local write "chunks"(w278) -> ()
    n133 = Unbundle By Name(w260) -> ("status"=w298:bool)
    n134 = Subtract(x=w269, y=w268) -> (x-y=w276:dbl)
    n135 = local write "progress (sec)"(w276) -> ()
    n136 = Compound Arithmetic op=OR("stop", w298) -> (w309:bool)
  }
  "Loop counter" <- w114
  "DO array  making time" <- w84
  "DO write time, ms" <- w83
  n137 = Increment(x=w114) -> (x+1=w110:i32)
  n138 = Divide(x=w110, y=w115) -> (x/y=w118:dbl)
  n139 = Multiply(x=w118, y=100.0) -> (x*y=w116:dbl)
  n140 = local write "Progress, %"(w116) -> ()
  n141 = disable-structure shown="Disabled" {
    frame Disabled {
      n142 = Unbundle By Name() -> ("Lockin mode"=w318:enum16{"SRS", "NI-DAQ"})  [unwired: 1 in]
      n143 = case shown="\"NI-DAQ\"" w318 {
        tunnel: [_ w320] -> _
        tunnel: [_ w319] -> _
        frame "SRS", Default {
        }
        frame "NI-DAQ" {
          # "Download freq array"
          n144 = call "ProgramFreqBulk.vi"() -> ("error out"=w320:errorcluster, "RUS settings out"=w319:T11)  [unwired: 5 in, 5 out]
        }
      }
    }
    frame Enabled {
    }
  }
  n145 = Array Subset(array=w62, length=w61) -> (w45:dbl[])  [unwired: 1 in]
  n146 = Array Subset(array=w106, length=w61) -> (w71:cdb[])  [unwired: 1 in]
  n147 = disable-structure shown="Disabled" {
    frame Disabled {
      n148 = while {
        shift-right: [w324] -> _
        shift-left: _ -> [w325]
        shift-right: [w323] -> _
        shift-left: _ -> [w326]
        tunnel: [w321] -> _
        stop <- TRUE stop-if-true
        n149 = property class="DAQmx Write"(reference=w325, error in=w326) -> (reference out=w324:refnum<k21>, error out=w323:errorcluster, "SpaceAvail"=w321:u32)
      }
    }
    frame Enabled {
    }
  }
  n150 = call "single sweep - rus clean up.vi"("Zero amplitude at the end"="Zero amplitude at the end", "Stop user event"=w64, "error in (no error)"=w23, "RUS settings"=w63) -> ("error out"=w100:errorcluster, "STD status byte"=→"STD status byte":u8, "Error status byte\n(bit 5 - FAST aborted)"=→"Error status byte\n(bit 5 - FAST aborted)":u8, "RUS settings out"=w95:T11)  [unwired: 4 in]
  n151 = Complex To Re/Im(x + iy=w71) -> (x=w70:dbl[], y=w69:dbl[])
  n152 = Not(x=w105) -> (.not. x?=w93:bool)
  n153 = disable-structure shown="Enabled" {
    disable-tunnel: w69 -> [w331 w333]
    disable-tunnel: w70 -> [w330 w332]
    disable-tunnel: [w329 w332] -> w67
    disable-tunnel: [w328 w333] -> w66
    disable-tunnel: w103 -> [w327 _]
    frame Disabled {
      n154 = call "Rotate Lockin Phase.vi"("Phase"=w327, "Array Y in"=w331, "Array X in"=w330) -> ("Array Y out"=w328:dbl[], "Array X out"=w329:dbl[])  [unwired: 7 out]
    }
    frame Enabled {
    }
  }
  n155 = case shown="True" w93 {
    tunnel: w100 -> [w334 w341]
    tunnel: [w334 w339] -> w120
    tunnel: w71 -> [_ w335]
    tunnel: w95 -> [_ w338]
    tunnel: w45 -> [_ w336]
    frame False {
    }
    frame True {
      n156 = call "single sweep - save rus data.vi"("write freq in"="saved frequency unit", "error in (no error)"=w341, "rus response"=w335, "F Array"=w336, "RUS settings"=w338) -> ("error out"=w339:errorcluster, "Actual file path"=→"Actual file path":path)  [unwired: 5 in]
    }
  }
  n157 = Divide(x=w45, y=1000 ("dimension size")) -> (x/y=w44:dbl[])
  n158 = Bundle(w67, w66) -> (w68:cluster{dbl[], dbl[]})  [unwired: 1 out]
  n159 = Bundle(w44, w67) -> (w109:cluster{dbl[], dbl[]})  [unwired: 1 out]
  n160 = Bundle(w44, w66) -> (w108:cluster{dbl[], dbl[]})  [unwired: 1 out]
  n161 = Build Array(w109, w108) -> (w72:cluster{dbl[], dbl[]}[])
  n162 = Build Array(w68) -> (w65:cluster{dbl[], dbl[]}[])
  n163 = local write "Plot:complex plane"(w65) -> ()
  n164 = local write "Plot:response"(w72) -> ()
  n165 = case shown="True" "Bypass error dialog" {
    tunnel: [w343 w345] -> w123
    tunnel: w120 -> [w342 w345]
    frame False {
      w344 = T16 3 items=["no dialog", "OK message", "continue or stop message", "OK message + warnings", "continue/stop + warnings"] ("type of dialog (OK msg:1)")
      n166 = call <vilib>:"General Error Handler.vi"("type of dialog (OK msg:1)"=w344, "error in (no error)"=w342) -> ("error out"=w343:errorcluster)  [unwired: 13 out]
    }
    frame True {
    }
  }
  "error out" <- w123
